vi "Check and compute displacements.vi"(8 "error in (no error)":errorcluster, 11 "Retiga in":refnum<class "Retiga.lvclass">) -> (0 "error out":errorcluster, 1 "fine?":bool, 2 "translation out":dbl[unit], 3 "Retiga out":refnum<class "Retiga.lvclass">)   [LabVIEW 2012, in "Retiga.lvclass"]
uses:
  Retiga.lvclass
  dependencies/ImageReg/Registration method.ctl
  Retiga.lvclass/Retiga.ctl
  <vilib>/Analysis/baseanly.llb/Mean (DBL).vi
  <vilib>/Analysis/NI_AALBase.lvlib
  <vilib>/gmath/NI_Gmath.lvlib
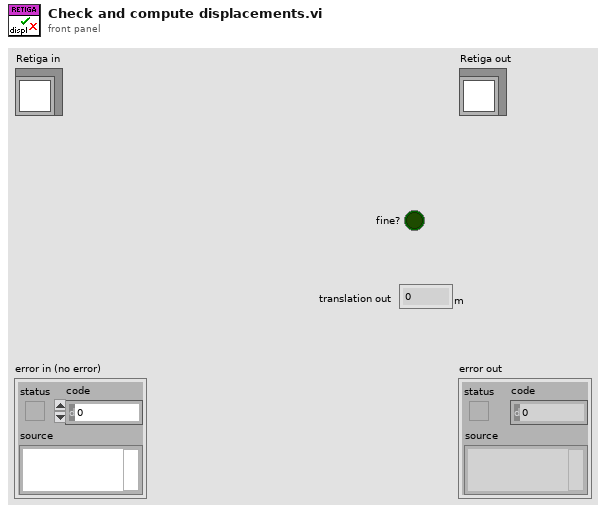
[diagram p1: front panel]
types:
  T1 = typedef "Registration method.ctl" = enum16{"Binarization", "Difference of Gaussians", "Edges Detection", "Gaussians and Binarization", "Edges and Gaussians", "Edges and Binarization", "All"}
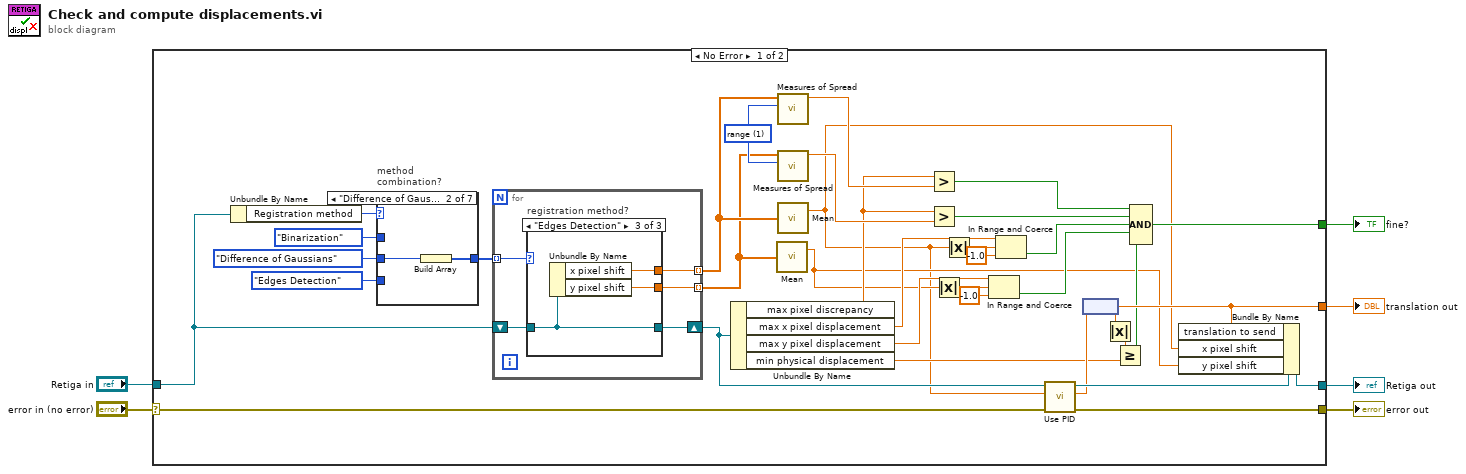
[diagram p0: block diagram]
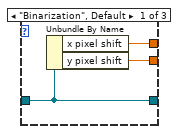
[diagram p2: hidden frame]
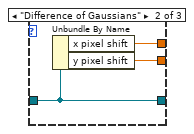
[diagram p3: hidden frame]
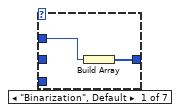
[diagram p4: hidden frame]
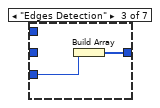
[diagram p5: hidden frame]
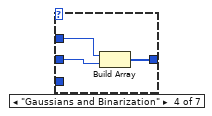
[diagram p6: hidden frame]
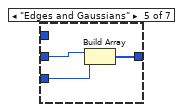
[diagram p7: hidden frame]
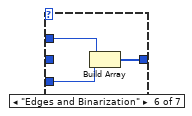
[diagram p8: hidden frame]
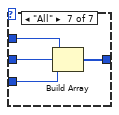
[diagram p9: hidden frame]
diagram:
  n1 = case shown="No Error" "error in (no error)" {
    selector: "error in (no error)" -> [w17 w76]
    tunnel: [w16 w76] -> w5
    tunnel: [w14 w75] -> w3
    tunnel: "Retiga in" -> [w28 w75]
    tunnel: [w13 _] -> w2
    tunnel: [w39 _] -> w1
    frame No Error {
      w26 = 1 items=["standard deviation", "range", "mean absolute deviation", "interquartile range"] ("type")
      n2 = Unbundle By Name(w28) -> ("Registration method"=w30:T1)
      n3 = case "method\ncombination?" shown="\"Difference of Gaussians\"" w30 {
        tunnel: [w57 w59 w61 w64 w67 w70 w74] -> w29
        tunnel: Registration_method."Difference of Gaussians" ("Registration method") -> [_ w58 _ w62 w66 _ w71]
        tunnel: Registration_method."Binarization" ("Registration method") -> [w56 _ _ w63 _ w68 w73]
        tunnel: Registration_method."Edges Detection" ("Registration method") -> [_ _ w60 _ w65 w69 w72]
        frame "Binarization", Default {
          n4 = Build Array(w56) -> (w57:T1[])
        }
        frame "Difference of Gaussians" {
          n5 = Build Array(w58) -> (w59:T1[])
        }
        frame "Edges Detection" {
          n6 = Build Array(w60) -> (w61:T1[])
        }
        frame "Gaussians and Binarization" {
          n7 = Build Array(w63, w62) -> (w64:T1[])
        }
        frame "Edges and Gaussians" {
          n8 = Build Array(w66, w65) -> (w67:T1[])
        }
        frame "Edges and Binarization" {
          n9 = Build Array(w68, w69) -> (w70:T1[])
        }
        frame "All" {
          n10 = Build Array(w73, w71, w72) -> (w74:T1[])
        }
      }
      n11 = for {
        tunnel: w29 -> [w46] mode=indexing
        shift-right: [w44] -> w18
        shift-left: w28 -> [w45]
        tunnel: [w43] -> w27 mode=indexing
        tunnel: [w42] -> w25 mode=indexing
        n12 = case "registration method?" shown="\"Edges Detection\"" w46 {
          tunnel: w45 -> [w49 w52 w55]
          tunnel: [w49 w52 w55] -> w44
          tunnel: [w48 w51 w54] -> w43
          tunnel: [w47 w50 w53] -> w42
          frame "Binarization", Default {
            n13 = Unbundle By Name(w49) -> ("x pixel shift"=w48:dbl, "y pixel shift"=w47:dbl)
          }
          frame "Difference of Gaussians" {
            n14 = Unbundle By Name(w52) -> ("x pixel shift"=w51:dbl, "y pixel shift"=w50:dbl)
          }
          frame "Edges Detection" {
            n15 = Unbundle By Name(w55) -> ("x pixel shift"=w54:dbl, "y pixel shift"=w53:dbl)
          }
        }
      }
      n16 = Unbundle By Name(w18) -> ("max pixel discrepancy"=w21:dbl, "max x pixel displacement"=w20:dbl, "max y pixel displacement"=w19:dbl, "min physical displacement"=w11:dbl[unit])
      n17 = call-poly <vilib>:"Mean.vi"("X"=w25) -> ("mean"=w8:dbl)  [unwired: 1 out]
      n18 = call <vilib>:"Measures of Spread.vi"("type"=w26, "x array"=w27) -> ("spread value"=w24:dbl)  [unwired: 8 in, 1 out]
      n19 = call <vilib>:"Measures of Spread.vi"("type"=w26, "x array"=w25) -> ("spread value"=w23:dbl)  [unwired: 8 in, 1 out]
      n20 = call-poly <vilib>:"Mean.vi"("X"=w27) -> ("mean"=w7:dbl)  [unwired: 1 out]
      n21 = Greater?(x=w21, y=w24) -> (0:w34:bool)
      n22 = Greater?(x=w21, y=w23) -> (0:w22:bool)
      n23 = Absolute Value(x=w8) -> (abs(x)=w38:dbl)
      n24 = Absolute Value(x=w7) -> (abs(x)=w40:dbl)
      n25 = In Range and Coerce(upper limit=w19, x=w38, lower limit=-1.0) -> (In Range?=w10:bool)  [unwired: 1 out]
      n26 = In Range and Coerce(upper limit=w20, x=w40, lower limit=-1.0) -> (In Range?=w41:bool)  [unwired: 1 out]
      n27 = call-dynamic "Use PID.vi"("error in (no error)"=w17, "X pixel translation"=w7, "Retiga in"=w18) -> ("error out"=w16:errorcluster, "translation out"=w12:dbl, "Retiga out"=w15:refnum<class "Retiga.lvclass">)  [unwired: 6 in]
      n28 = node(w12) -> (w13:dbl[unit])
      n29 = Absolute Value(x=w13) -> (abs(x)=w35:dbl[unit])
      n30 = Greater Or Equal?(x=w35, y=w11) -> (x >= y?=w9:bool)
      n31 = Compound Arithmetic op=AND(w34, w22, w41, w10, w9) -> (w39:bool)
      n32 = Bundle By Name(cluster=w15, "translation to send"=w13, "x pixel shift"=w7, "y pixel shift"=w8) -> (w14:refnum<class "Retiga.lvclass">)
    }
    frame Error {
    }
  }
  "error out" <- w5
  "Retiga out" <- w3
  "fine?" <- w1
  "translation out" <- w2
